vi "Test-Global2.vi"() -> ()   [LabVIEW 2014]
uses:
  Terminal-Global-SetValues.vi
panel:
  out "输入数值":dbl
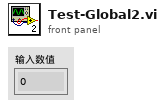
[diagram p1: front panel]
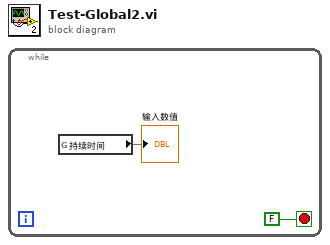
[diagram p0: block diagram]
diagram:
  n1 = while {
    stop <- FALSE stop-if-true
    n2 = global read "Terminal-Global-SetValues.vi" "持续时间"() -> (→"输入数值")
  }
